vi "Get Last.vi"(0 "Subroutine in":refnum<class "Subroutine.lvclass">, 1 "Linked List Ref":refnum<data-value>, 5 "Active Unique ID":string, 9 "Active Element Index":i32, 11 "error in (no error)":errorcluster) -> (3 "Linked List Ref out":refnum<data-value>, 4 "Executioner out":refnum<class "Executioner.lvclass">, 6 "Active Unique ID out":string, 10 "Active Element Index out":i32, 12 "Restore Point":bool, 13 "Complete":bool, 14 "Stop":bool, 15 "error out":errorcluster)   [LabVIEW 2020, in "Test Executive.lvlib" / "Subroutine.lvclass"]
uses:
  <vilib>/gpm_packages/@cs/test-executive/Source/Test Executive/Subroutine/Subroutine.lvclass
  C:/Program Files/National Instruments/LabVIEW 2020/vi.lib/gpm_packages/@cs/test-executive/Source/Test Executive/Executioner/Executioner.lvclass
  <vilib>/gpm_packages/@cs/test-executive/Source/Test Executive/Executioner/Executioner.lvclass
  <vilib>/gpm_packages/@cs/linked-list/Source/Linked List/ILinkedList/ILinked List.lvclass
  4fd378ea-8446-4c29-9057-0b9582e709d7.vi
  7a1b7c76-c447-4cbe-ba03-9c129f6599f4.vi
  <vilib>/gpm_packages/@cs/linked-list/Source/Linked List/Linked List Ref/Linked List Ref.lvclass
  e1a69301-650a-4345-9450-f58f2c381fc0.vi
  049bc9e2-7404-4dee-baf6-27a84f02d5ca.vi
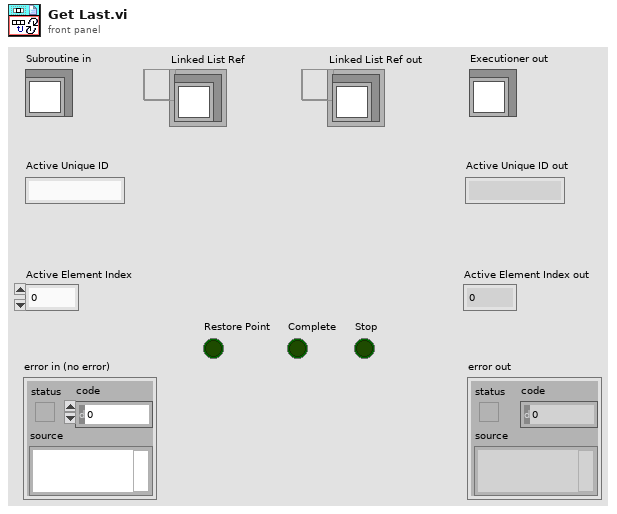
[diagram p1: front panel]
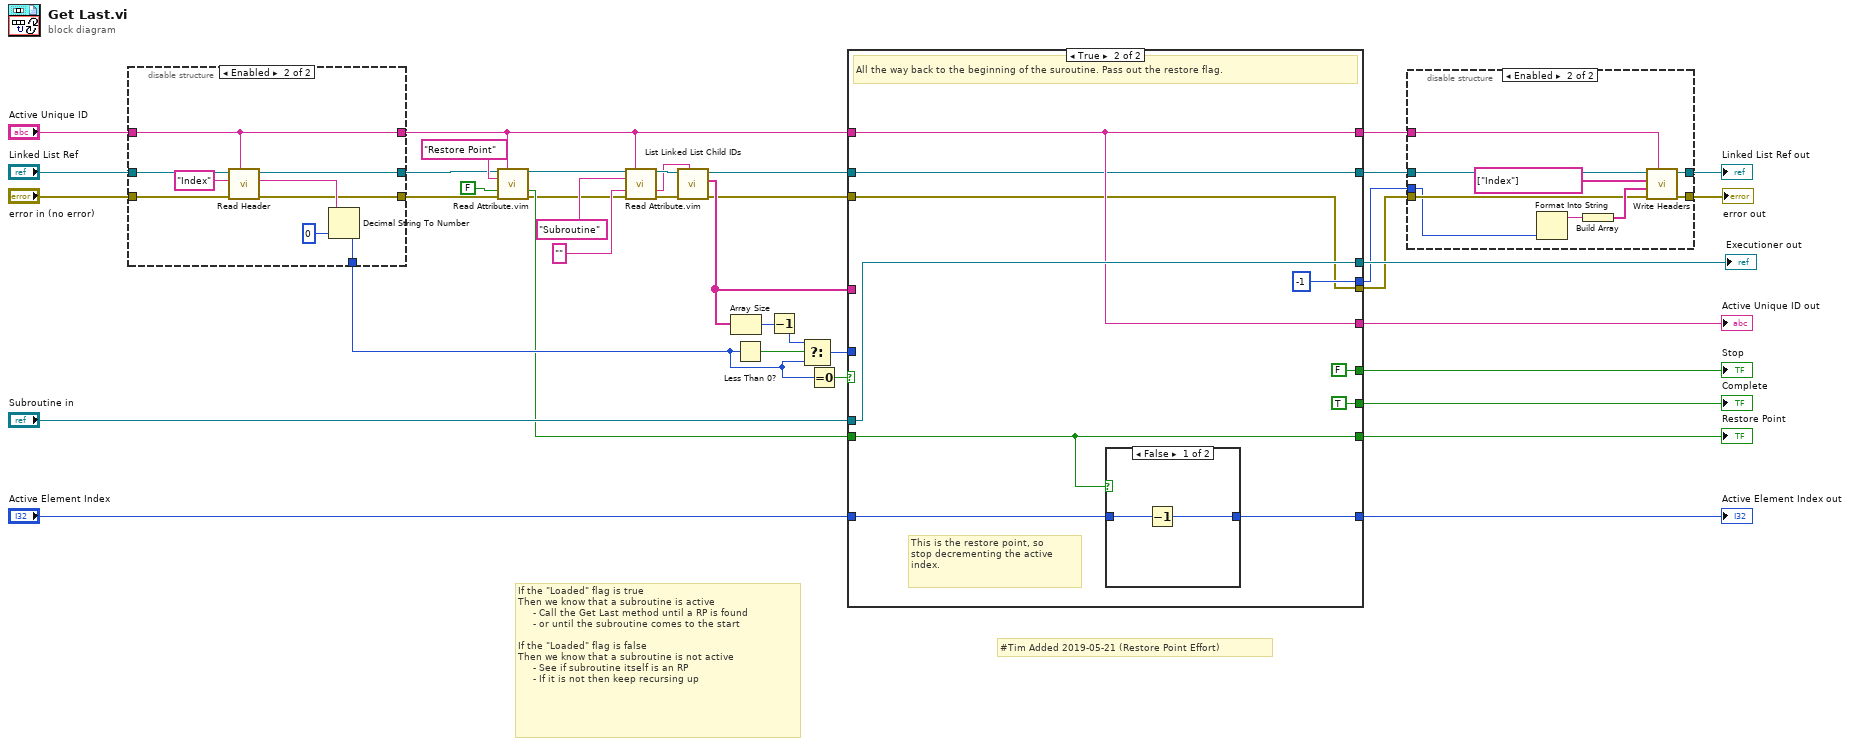
[diagram p0: block diagram]
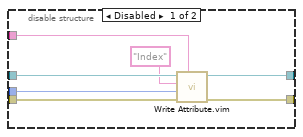
[diagram p2: hidden frame]
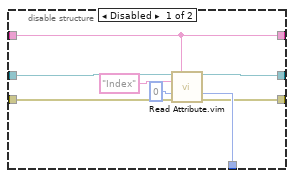
[diagram p3: hidden frame]
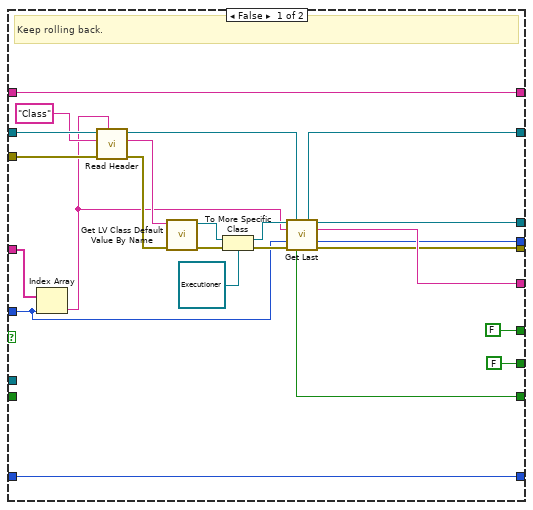
[diagram p4: hidden frame]
diagram:
  # "If the \"Loaded\" flag is true\nThen we know that a subroutine is active\n     - Call the Get Last method until a RP is found\n     - or until the subroutine comes to the start\n\nIf the \"Loaded\" flag is false\nThen we know that a subroutine is not active\n     - See if subroutine itself is an RP\n     - If it is not then keep recursing up"
  # "#Tim Added 2019-05-21 (Restore Point Effort)"
  n1 = disable-structure shown="Enabled" {
    disable-tunnel: "Linked List Ref" -> [w47 w53]
    disable-tunnel: "error in (no error)" -> [w44 w51]
    disable-tunnel: [w43 w49] -> w29
    disable-tunnel: [w42 w52] -> w14
    disable-tunnel: [w41 w50] -> w13
    disable-tunnel: "Active Unique ID" -> [w40 w48]
    disable-tunnel: [w40 w48] -> w1
    frame Disabled {
      n2 = call "Read Attribute.vim"("Linked List Ref"=w47, "Linked List ID"=w40, "Attribute Name"="Index", "Type"=0, "error in (no error)"=w44) -> ("Linked List Ref out"=w42:refnum<data-value>, "Attribute"=w43:i32, "error out"=w41:errorcluster)  [unwired: 5 in, 3 out]
    }
    frame Enabled {
      n3 = call <vilib>:"Read Header.vi"("Linked List ID"=w48, "error in (no error)"=w51, "Header Name"="Index" ("Attribute Name"), "Linked List Ref"=w53) -> ("error out"=w50:errorcluster, "Header Value"=w55:string, "Linked List Ref out"=w52:refnum<data-value>)  [unwired: 4 in, 1 out]
      n4 = Decimal String To Number(string=w55, default (0L)=0 ("Attribute")) -> (number=w49:i32)  [unwired: 1 in, 1 out]
    }
  }
  n5 = call "Read Attribute.vim"("Linked List Ref"=w14, "Linked List ID"=w1, "Attribute Name"="Restore Point", "Type"=FALSE, "error in (no error)"=w13) -> ("Linked List Ref out"=w9:refnum<data-value>, "Attribute"=w12:bool, "error out"=w6:errorcluster)  [unwired: 5 in, 3 out]
  n6 = call "Read Attribute.vim"("Linked List Ref"=w9, "Linked List ID"=w1, "Attribute Name"="Subroutine", "Type"="", "error in (no error)"=w6) -> ("Linked List Ref out"=w8:refnum<data-value>, "Attribute"=w4:string, "error out"=w7:errorcluster)  [unwired: 5 in, 3 out]
  n7 = call <vilib>:"List Linked List Child IDs.vi"("Linked List ID"=w4, "error in (no error)"=w7, "Linked List Ref"=w8) -> ("error out"=w27:errorcluster, "Child IDs"=w28:string[], "Linked List Ref out"=w35:refnum<data-value>)  [unwired: 6 in]
  n8 = Array Size(array=w28) -> (size(s)=w34:i32)
  n9 = Less Than 0?(x=w29) -> (x < 0?=w33:bool)
  n10 = Decrement(x=w34) -> (x-1=w32:i32)
  n11 = Select(t=w32, s=w33, f=w29) -> (s? t:f=w31:i32)
  n12 = Equal To 0?(x=w29) -> (x = 0?=w30:bool)
  n13 = case shown="True" w30 {
    tunnel: w35 -> [w79 w83]
    tunnel: w31 -> [w70 _]
    tunnel: w28 -> [w80 _]
    tunnel: w27 -> [w77 w82]
    tunnel: "Active Element Index" -> [w69 w86]
    tunnel: [w69 w85] -> w25
    tunnel: "Subroutine in" -> [_ w89]
    tunnel: [w67 w83] -> w20
    tunnel: [w64 w84] -> w23
    tunnel: [w63 w89] -> w22
    tunnel: w1 -> [w62 w84]
    tunnel: [w62 w84] -> w19
    tunnel: [w61 w82] -> w18
    tunnel: [w60 w81] -> w21
    tunnel: [w59 -1 ("Active Element Index out")] -> w17
    tunnel: [FALSE ("Complete") TRUE ("Complete")] -> w16
    tunnel: [FALSE ("Complete") FALSE ("Complete")] -> w15
    tunnel: w12 -> [_ w81]
    frame False {
      # "Keep rolling back."
      n14 = Index Array(array=w80, index=w70) -> (element=w65:string)
      n15 = call <vilib>:"Read Header.vi"("Linked List ID"=w65, "error in (no error)"=w77, "Header Name"="Class", "Linked List Ref"=w79) -> ("error out"=w75:errorcluster, "Header Value"=w76:string, "Linked List Ref out"=w68:refnum<data-value>)  [unwired: 4 in, 1 out]
      n16 = call <vilib>:"Get LV Class Default Value By Name.vi"("error in (no error)"=w75, "class name"=w76) -> ("error out"=w74:errorcluster, "object"=w73:refnum<class>)  [unwired: 8 in]
      n17 = To More Specific Class(target class=refnum<class "Executioner.lvclass"> refnum ("Test Executive.lvlib:Executioner.lvclass"), reference=w73, error in=w74) -> (specific class reference=w66:refnum<class "Executioner.lvclass">, error out=w71:errorcluster)
      n18 = call-dynamic "Get Last.vi"("Executioner in"=w66, "Linked List Ref"=w68, "Active Unique ID"=w65, "Active Element Index"=w70, "error in (no error)"=w71) -> ("Linked List Ref out"=w67:refnum<data-value>, "Executioner out"=w63:refnum<class "Executioner.lvclass">, "Active Unique ID out"=w64:string, "Active Element Index out"=w59:i32, "Restore Point"=w60:bool, "error out"=w61:errorcluster)  [unwired: 3 in, 2 out]
    }
    frame True {
      # "This is the restore point, so\nstop decrementing the active\nindex."
      # "All the way back to the beginning of the suroutine. Pass out the restore flag."
      n19 = case shown="False" w81 {
        tunnel: w86 -> [w92 w93]
        tunnel: [w91 w93] -> w85
        frame False {
          n20 = Decrement(x=w92) -> (x-1=w91:i32)
        }
        frame True {
        }
      }
    }
  }
  "Executioner out" <- w22
  "Active Unique ID out" <- w23
  "Active Element Index out" <- w25
  "Restore Point" <- w21
  "Complete" <- w16
  "Stop" <- w15
  n21 = disable-structure shown="Enabled" {
    disable-tunnel: w20 -> [w100 w106]
    disable-tunnel: w19 -> [w99 w102]
    disable-tunnel: w18 -> [w97 w103]
    disable-tunnel: w17 -> [w96 w101]
    disable-tunnel: [w95 w105] -> w3
    disable-tunnel: [w94 w104] -> w2
    frame Disabled {
      n22 = call "Write Attribute.vim"("Linked List ID"=w99, "error in (no error)"=w97, "Attribute"=w96, "Attribute Name"="Index", "Linked List Ref"=w100) -> ("error out"=w94:errorcluster, "Linked List Ref out"=w95:refnum<data-value>)  [unwired: 3 in, 2 out]
    }
    frame Enabled {
      n23 = Format Into String(w101) -> (resulting string=w108:string)  [unwired: 3 in, 1 out]
      n24 = Build Array(w108) -> (w107:string[])
      n25 = call <vilib>:"Write Headers.vi"("Linked List ID"=w102, "error in (no error)"=w103, "Header Values"=w107, "Header Names"=string[] ["Index"], "Linked List Ref"=w106) -> ("error out"=w104:errorcluster, "Linked List Ref out"=w105:refnum<data-value>)  [unwired: 5 in]
    }
  }
  "error out" <- w2
  "Linked List Ref out" <- w3
